vi "users update current user header.vi"(8 "error in (no error)":errorcluster, 9 "Current User Changes? (f)":bool, 10 "new Current User":T1, 11 "HTTP header (\"\")":string) -> (0 "error out":errorcluster, 3 "updated HTTP header":string)   [LabVIEW 2011]
uses:
  server/database/Users/User Record.ctl
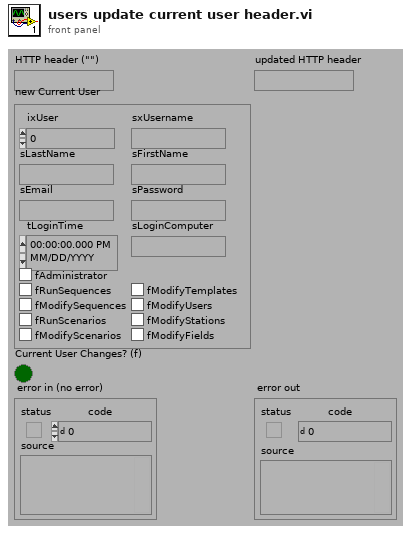
[diagram p1: front panel]
types:
  T1 = typedef "User Record.ctl" = cluster{"ixUser":i32, "sxUsername":string, "sLastName":string, "sFirstName":string, "sEmail":string, "sPassword":string, "tLoginTime":timestamp, "sLoginComputer":string, "fAdministrator":bool, "fRunSequences":bool, "fModifySequences":bool, "fRunScenarios":bool, "fModifyScenarios":bool, "fModifyTemplates":bool, "fModifyUsers":bool, "fModifyStations":bool, "fModifyFields":bool}
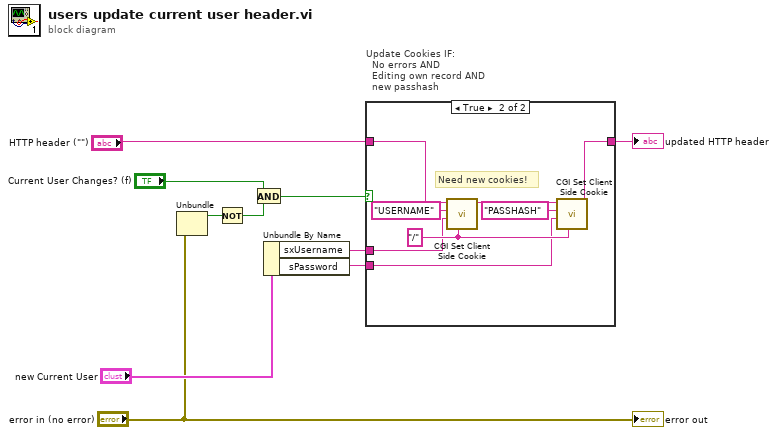
[diagram p0: block diagram]
diagram:
  n1 = Unbundle("error in (no error)") -> ("status"=w5:bool)  [unwired: 2 out]
  n2 = Not(x=w5) -> (.not. x?=w4:bool)
  n3 = And(x="Current User Changes? (f)", y=w4) -> (x .and. y?=w6:bool)
  n4 = Unbundle By Name("new Current User") -> ("sxUsername"=w10:string, "sPassword"=w9:string)
  n5 = case "Update Cookies IF:\n  No errors AND\n  Editing own record AND\n  new passhash" shown="True" w6 {
    tunnel: [w11 w14] -> w7
    tunnel: "HTTP header (\"\")" -> [w11 w15]
    tunnel: w10 -> [_ w13]
    tunnel: w9 -> [_ w12]
    frame False {
    }
    frame True {
      w16 = "/"
      # "Need new cookies!"
      n6 = call "CGI Set Client Side Cookie.vi"("path (\"\")"=w16, "cookie value"=w13, "cookie name"="USERNAME", "header in"=w15) -> ("header out"=w19:string)  [unwired: 1 in, 6 out]
      n7 = call "CGI Set Client Side Cookie.vi"("path (\"\")"=w16, "cookie value"=w12, "cookie name"="PASSHASH", "header in"=w19) -> ("header out"=w14:string)  [unwired: 1 in, 6 out]
    }
  }
  "updated HTTP header" <- w7
  "error out" <- "error in (no error)"
